vi "Add DataColumns to DataTable.vi"(8 "错误输入（无错误）":errorcluster, 10 "DataColumns":refnum<k24>[](array[refnum]), 11 "DataTable":refnum<k24>) -> (0 "错误输出":errorcluster, 3 "DataTable Out":refnum<k24>)   [LabVIEW 2012, in "DataGridView.lvlib"]
uses:
  DataGridView.lvlib
  System.Data
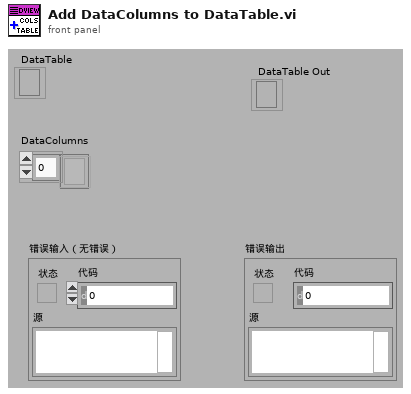
[diagram p1: front panel]
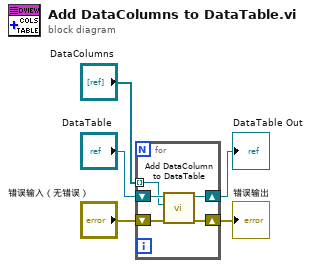
[diagram p0: block diagram]
diagram:
  n1 = for {
    shift-right: [w8] -> w2
    shift-left: "DataTable" -> [w10]
    tunnel: "DataColumns" -> [w7] mode=indexing
    shift-right: [w6] -> w1
    shift-left: "错误输入（无错误）" -> [w9]
    n2 = call "Add DataColumn to DataTable.vi"("错误输入（无错误）"=w9, "DataColumn"=w7, "DataTable"=w10) -> ("错误输出"=w6:errorcluster, "DataTable"=w8:refnum<k24>)  [unwired: 7 in]
  }
  "DataTable Out" <- w2
  "错误输出" <- w1
